vi "Create.vi"(8 "error in (no error)":errorcluster, 10 "Barcode Content":string) -> (0 "error out":errorcluster, 3 "Barcode Reader out":refnum<class "Barcode Reader.lvclass">)   [LabVIEW 2020, in "Barcode Reader First Iteration.lvlib" / "Barcode Reader.lvclass"]
uses:
  Barcode Reader.lvclass
  Barcode Reader.lvclass/Barcode Reader.ctl
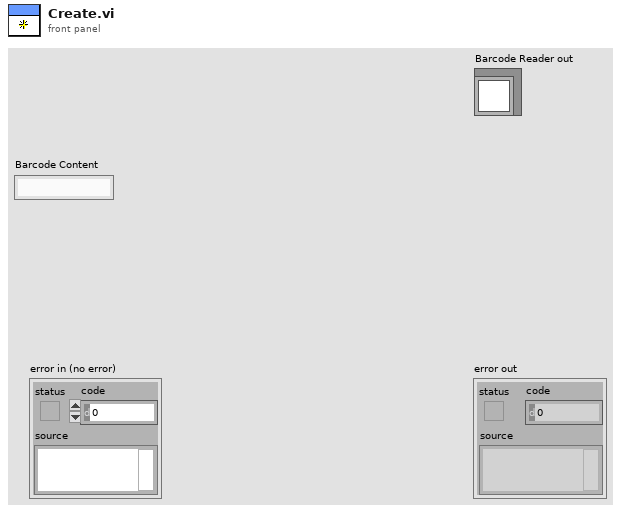
[diagram p1: front panel]
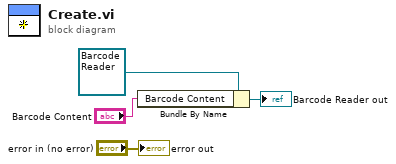
[diagram p0: block diagram]
diagram:
  n1 = Bundle By Name(cluster=refnum<class "Barcode Reader.lvclass"> refnum ("Barcode Reader in"), "Barcode Content"="Barcode Content") -> (→"Barcode Reader out":refnum<class "Barcode Reader.lvclass">)
  "error out" <- "error in (no error)"
